vi "Build core.vi"(6 "Previous Build's Artifacts":refnum<class "Build Artifact.lvclass">[](array[class]), 7 "Progress":refnum<class "Progress.lvclass">, 8 "error in (no error)":errorcluster, 10 "Build Cache":refnum<class "Build Cache.lvclass">, 11 "Build Item in":refnum<class "Build Package Step.lvclass">) -> (0 "error out":errorcluster, 1 "Explore Path":path, 2 "Build Results":T1, 4 "New Artifacts":refnum<class "Build Artifact.lvclass">[](array[class]))   [LabVIEW 2019, in "VIPM.lvlib" / "Build Package Step.lvclass"]
doc: "Performs all the necessary build actions for the build step.\n\nCopyright: MGI 2016\nAuthor: Derek Trepanier"
uses:
  Build Package Step.lvclass
  libs/Solution.lvlibp/Solution/Progress/Progress.lvclass
  libs/Solution.lvlibp/Solution/Build Artifact/Build Artifact.lvclass
  libs/Solution.lvlibp/Solution/Build Item/Build Result.ctl
  libs/Solution.lvlibp/Solution/Build Cache/Build Cache.lvclass
  Build Package Step.lvclass/Build Package Step.ctl
  libs/Project.lvlibp/Project/Binary File/Binary File.lvclass
  C:/Users/pasca/source/repos/mgi-solution-explorer-extensions/libs/Solution.lvlibp/Solution/Build Artifact/Build Artifact.lvclass
  <vilib>/JKI/VIPM API/VIPM API_vipm_api.lvlib
  libs/Solution.lvlibp/Solution/Build Item/Build Step.lvclass
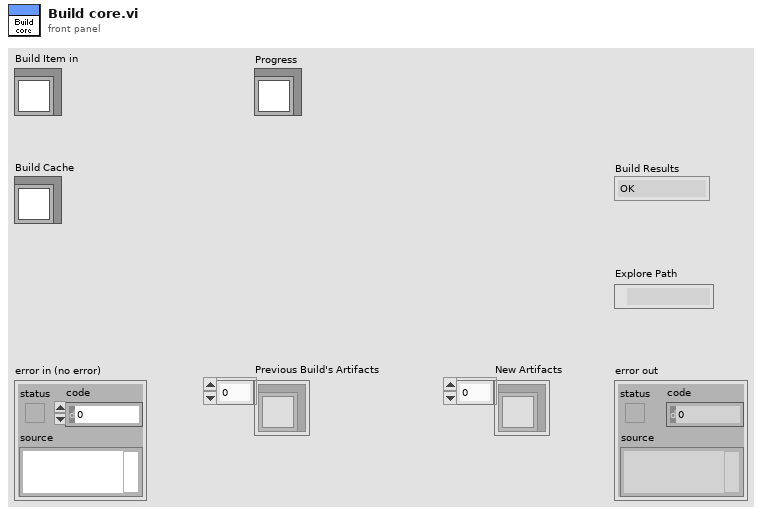
[diagram p1: front panel]
types:
  T1 = typedef "Solution.lvlibp/Build Step.lvclass/Build Result.ctl" = enum16{"OK", "Skipped", "Error"}
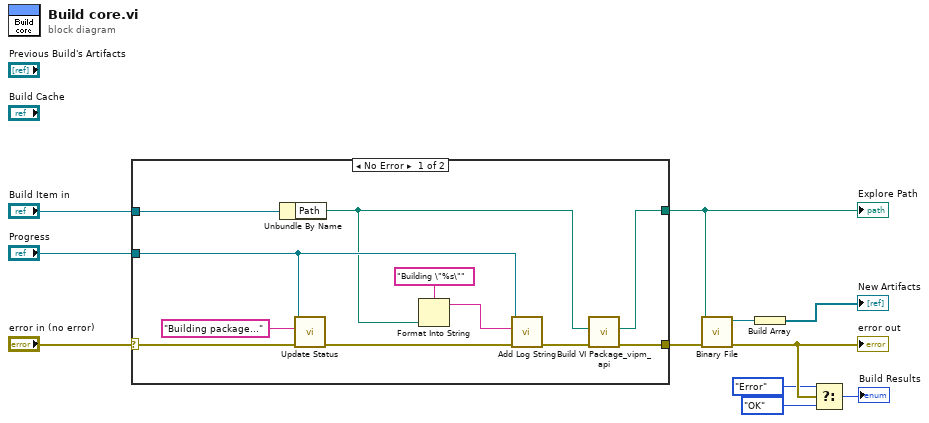
[diagram p0: block diagram]
diagram:
  n1 = case shown="No Error" "error in (no error)" {
    selector: "error in (no error)" -> [w21 w23]
    tunnel: [w12 w23] -> w10
    tunnel: [w13 _] -> w9
    tunnel: "Build Item in" -> [w22 _]
    tunnel: "Progress" -> [w17 _]
    frame No Error {
      n2 = Unbundle By Name(w22) -> ("Path"=w14:path)
      n3 = call "Update Status.vi"("error in (no error)"=w21, "Status String"="Building package...", "Progress in"=w17) -> ("error out"=w19:errorcluster)  [unwired: 8 in]
      n4 = Format Into String(format string="Building \"%s\"" ("Log Item"), w14) -> (resulting string=w16:string)  [unwired: 2 in, 1 out]
      n5 = call "Add Log String.vi"("error in (no error)"=w19, "Log Item"=w16, "Progress in"=w17) -> ("error out"=w18:errorcluster)  [unwired: 8 in]
      n6 = call <vilib>:"Build VI Package_vipm_api.vi"("error in (no error)"=w18, "Path to VIPB File"=w14) -> ("error out"=w12:errorcluster, "Build Output"=w13:path)  [unwired: 8 in]
    }
    frame Error {
    }
  }
  "Explore Path" <- w9
  n7 = call "Binary File.vi"("error in (no error)"=w10, "File"=w9) -> ("error out"=w3:errorcluster, "Binary File out"=w8:refnum<class "Binary File.lvclass">)  [unwired: 8 in]
  "error out" <- w3
  n8 = Build Array(w8) -> (→"New Artifacts":refnum<class "Binary File.lvclass">[])
  n9 = Select(t=Build_Result."Error" ("Build Results"), s=w3, f=Build_Result."OK" ("Build Results")) -> (s? t:f=→"Build Results":T1)
